vi "INIT AIR.vi"(8 "error in (no error)":errorcluster) -> (0 "error out":errorcluster)   [LabVIEW 2023]
uses:
  Global INIT.vi
  <vilib>/Rock Robotics/WPI/Utilities/WPI_GetSetVariantRefNum.vi
  <vilib>/Rock Robotics/WPI/Solenoid/WPI_SolenoidOpenSingle.vi
  <vilib>/Rock Robotics/WPI/Solenoid/WPI_SolenoidOpenDouble.vi
  <vilib>/Rock Robotics/WPI/Solenoid/WPI_SolenoidSetEnum.vi
panel:
  in  "Pneumatics device (def)":u8=2
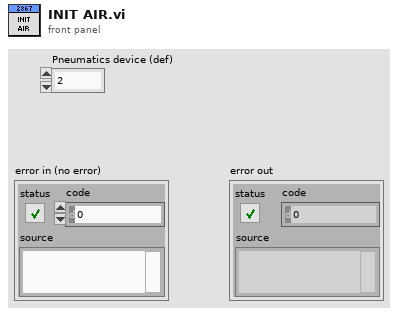
[diagram p1: front panel]
types:
  T1 = typedef "ctrl compressor begin.ctl" = cluster{"description":string, "Installed?":bool, "refnum name":string, "Feedback Configuration":T2}
  T2 = typedef "ctrl compressor config.ctl" = cluster{"Feedback Sensor":T3, "Max Pressure (PSI)":dbl, "Min Pressure (PSI)":dbl}
  T3 = typedef "WPI_CompressorFeedbackMode.ctl" = enum16{"Analog Only", "Digital Only", "Hybrid"}
  T4 = typedef "ctrl solenoid.ctl" = cluster{"description":string, "Installed?":bool, "refnum name":string, "coils":enum16{"Single", "Double"}, "forward channel":T5, "reverse channel":T5, "initial value":T6}
  T5 = typedef "WPI_SolenoidChannel.ctl" = enum8{"Solenoid 0", "Solenoid 1", "Solenoid 2", "Solenoid 3", "Solenoid 4", "Solenoid 5", "Solenoid 6", "Solenoid 7", "Solenoid 8", "Solenoid 9", "Solenoid 10", "Solenoid 11", "Solenoid 12", "Solenoid 13", "Solenoid 14", "Solenoid 15", "Invalid"}
  T6 = typedef "WPI_SolenoidValue.ctl" = enum16{"Off", "On", "Forward", "Reverse"}
  T7 = typedef "WPI_SolenoidDevRef.ctl" = cluster{"DevStatus":errorcluster, "Pneumatics Control Module":u8, "Forward Solenoid Channel":T5, "Reverse Solenoid Channel":T5}
  T8 = typedef "WPI_CompressorDevRef.ctl" = cluster{"DevStatus":errorcluster, "Pneumatics Control Module":u8}
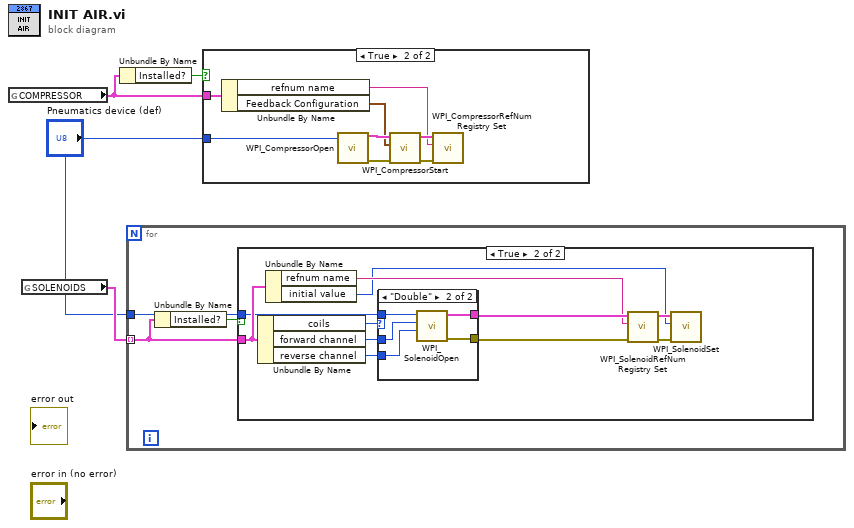
[diagram p0: block diagram]
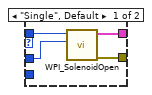
[diagram p3: hidden frame]
diagram:
  n1 = global read "Global INIT.vi" "COMPRESSOR"() -> (w4:T1)
  n2 = global read "Global INIT.vi" "SOLENOIDS"() -> (w2:T4[])
  n3 = Unbundle By Name(w4) -> ("Installed?"=w3:bool)
  n4 = for {
    tunnel: w2 -> [w6] mode=indexing
    tunnel: "Pneumatics device (def)" -> [w5]
    n5 = Unbundle By Name(w6) -> ("Installed?"=w7:bool)
    n6 = case shown="True" w7 {
      tunnel: w6 -> [_ w13]
      tunnel: w5 -> [_ w8]
      frame False {
      }
      frame True {
        n7 = Unbundle By Name(w13) -> ("coils"=w18:enum16{"Single", "Double"}, "forward channel"=w17:T5, "reverse channel"=w16:T5)
        n8 = Unbundle By Name(w13) -> ("refnum name"=w12:string, "initial value"=w9:T6)
        n9 = case shown="\"Double\"" w18 {
          tunnel: w17 -> [w22 w27]
          tunnel: w16 -> [_ w26]
          tunnel: [w20 w25] -> w14
          tunnel: [w21 w24] -> w15
          tunnel: w8 -> [w19 w23]
          frame "Single", Default {
            n10 = call-poly <vilib>:"WPI_SolenoidOpen.vi"("Solenoid Channel"=w22, "Pneumatics Device (def)"=w19) -> ("error out"=w21:errorcluster, "SolenoidDevRef"=w20:T7)  [unwired: 8 in]
          }
          frame "Double" {
            n11 = call-poly <vilib>:"WPI_SolenoidOpen.vi"("Reverse Solenoid Channel"=w26, "Forward Solenoid Channel"=w27, "Pneumatics Device (def)"=w23) -> ("error out"=w24:errorcluster, "SolenoidDevRef"=w25:T7)  [unwired: 7 in]
          }
        }
        n12 = call <vilib>:"WPI_SolenoidRefNum Registry Set.vi"("error in (no error)"=w15, "refnum name"=w12, "SolenoidDevRef"=w14) -> ("error out"=w11:errorcluster, "SolenoidDevRef"=w10:T7)  [unwired: 7 in]
        n13 = call-poly <vilib>:"WPI_SolenoidSet.vi"("error in (no error)"=w11, "Value"=w9, "SolenoidDevRef"=w10) -> ()  [unwired: 7 in, 2 out]
      }
    }
  }
  n14 = case shown="True" w3 {
    tunnel: w4 -> [_ w29]
    tunnel: "Pneumatics device (def)" -> [_ w28]
    frame False {
    }
    frame True {
      n15 = Unbundle By Name(w29) -> ("refnum name"=w31:string, "Feedback Configuration"=w30:T2)
      n16 = call <vilib>:"WPI_CompressorOpen.vi"("Pneumatics device (def)"=w28) -> ("CompressorDevRef"=w34:T8, "error out"=w35:errorcluster)  [unwired: 13 in]
      n17 = call <vilib>:"WPI_CompressorStart.vi"("error in (no error)"=w35, "Feedback Configuration"=w30, "CompressorDevRef"=w34) -> ("error out"=w33:errorcluster, "CompressorDevRef"=w32:T8)  [unwired: 7 in]
      n18 = call <vilib>:"WPI_CompressorRefNum Registry Set.vi"("error in (no error)"=w33, "refnum name"=w31, "CompressorDevRef"=w32) -> ()  [unwired: 7 in, 2 out]
    }
  }
